vi "anodicFitTest.vi"() -> ()   [LabVIEW 2018]
uses:
  <vilib>/Utility/file.llb/Read Delimited Spreadsheet (DBL).vi
panel:
  in  "iCorr":dbl=0.009000000000000001 step=0.001 format="%#_13g"
  out "return":dbl
  out "anodicElements":i32=115
  out "eCorr":dbl=-0.202
  out "intersects":i32
  out "anodicFitCoeffs":dbl[](array[numeric])=[-0.23570360753794362, -0.007154949128379092, 0.0, 0.0]
  out "anodicTraceCoeffs":dbl[](array[numeric])=[-0.21186227610841735, 0.0007290916455038351, 0.0, 0.0]
  in  "y2":dbl=-0.22000000000000003 step=0.01 format="%#_13g"
  in  "yData Filename":string="yData2"
  in  "xData Filename":string="xData2"
  out "error out":errorcluster
  out "MEASUREMENT":cluster{"XCoords":dbl[], "YCoords":dbl[]}[](graph)=[{"XCoords"=[1.108281, 0.885344, 0.732926, 0.625224, 0.543485, 0.479698, 0.42809, 0.384497, 0.350199, 0.321029, 0.296828, 0.273749, 0.255959, 0.241054, 0.227752, 0.21493, 0.202269, 0.193774, 0.184158, 0.177427, 0.168131, 0.162041, 0.156591, 0.150822, 0.143289, 0.138641, 0.133833, 0.129666, 0.124858, 0.119889, 0.116844, 0.112998, 0.109952, 0.104824, 0.103221, 0.099375, 0.09649, 0.093765, 0.09072, 0.088957, 0.086072, 0.083508, 0.080302, 0.07918, 0.077097, 0.074853, 0.071968, 0.069564, 0.068122, 0.066198, 0.064596, 0.06139, 0.060749, 0.059147, 0.056903, 0.055621, 0.053377, 0.052095, 0.050812, 0.049049, 0.045684, 0.044722, 0.044081, 0.04344, 0.040074, 0.038952, 0.037991, 0.036709, 0.036709, 0.033824, 0.03142, 0.0319, 0.029817, 0.027733, 0.027092, 0.02565, 0.02581, 0.022605, 0.021323, 0.021323, 0.019079, 0.019399, 0.016514, 0.015553, 0.014591, 0.012988, 0.012988, 0.010745, 0.009783, 0.008661, 0.009142, 0.006417, 0.006898, 0.005295, 0.002731, 0.00209, 7e-06, 0.000487, 0.000635, 0.001756, 0.00368, 0.004641, 0.005763, 0.006404, 0.007526, 0.008167, 0.008808, 0.008969, 0.010892, 0.012975, 0.012655, 0.013616, 0.013616, 0.016501, 0.018104, 0.017463, 0.019386, 0.020668, 0.023072, 0.023714, 0.023714, 0.026278, 0.0274, 0.028041, 0.028682, 0.029964, 0.029964, 0.031727, 0.032208, 0.034452, 0.034452, 0.034452, 0.036535, 0.036696, 0.037657, 0.038939, 0.040702, 0.040863, 0.042305, 0.042145, 0.04519, 0.04535, 0.046632, 0.046632, 0.049036, 0.048876, 0.049838, 0.050158, 0.05144, 0.053364, 0.053684, 0.055447, 0.054646, 0.05689, 0.057531, 0.058172, 0.059454, 0.059775, 0.061057, 0.062659, 0.06298, 0.064262, 0.066185, 0.066826, 0.067468, 0.068429, 0.06907, 0.070352, 0.071635, 0.071474, 0.073237, 0.07468, 0.073878, 0.074359, 0.076763, 0.075802, 0.079328, 0.079648, 0.079969, 0.081251, 0.082533, 0.083815, 0.084456, 0.085738, 0.087822, 0.087982, 0.089745, 0.089905, 0.090547, 0.09247, 0.093431, 0.094874, 0.095996, 0.097919, 0.09824, 0.09856, 0.099201, 0.099201, 0.100964, 0.099842, 0.101445, 0.103368, 0.105292, 0.10465, 0.105933, 0.104971, 0.106894, 0.109138, 0.109459, 0.109459, 0.111382], "YCoords"=[-0.298, -0.297, -0.296, -0.295, -0.294, -0.293, -0.292, -0.291, -0.29, -0.289, -0.288, -0.287, -0.286, -0.285, -0.284, -0.283, -0.282, -0.281, -0.28, -0.279, -0.278, -0.277, -0.276, -0.275, -0.274, -0.273, -0.272, -0.271, -0.27, -0.269, -0.268, -0.267, -0.266, -0.265, -0.264, -0.263, -0.262, -0.261, -0.26, -0.259, -0.258, -0.257, -0.256, -0.255, -0.254, -0.253, -0.252, -0.251, -0.25, -0.249, -0.248, -0.247, -0.246, -0.245, -0.244, -0.243, -0.242, -0.241, -0.24, -0.239, -0.238, -0.237, -0.236, -0.235, -0.234, -0.233, -0.232, -0.231, -0.23, -0.229, -0.228, -0.227, -0.226, -0.225, -0.224, -0.223, -0.222, -0.221, -0.22, -0.219, -0.218, -0.217, -0.216, -0.215, -0.214, -0.213, -0.212, -0.211, -0.21, -0.209, -0.208, -0.207, -0.206, -0.205, -0.204, -0.203, -0.202, -0.201, -0.2, -0.199, -0.198, -0.197, -0.196, -0.195, -0.194, -0.193, -0.192, -0.191, -0.19, -0.189, -0.188, -0.187, -0.186, -0.185, -0.184, -0.183, -0.182, -0.181, -0.18, -0.179, -0.178, -0.177, -0.176, -0.175, -0.174, -0.173, -0.172, -0.171, -0.17, -0.169, -0.168, -0.167, -0.166, -0.165, -0.164, -0.163, -0.162, -0.161, -0.16, -0.159, -0.158, -0.157, -0.156, -0.155, -0.154, -0.153, -0.152, -0.151, -0.15, -0.149, -0.148, -0.147, -0.146, -0.145, -0.144, -0.143, -0.142, -0.141, -0.14, -0.139, -0.138, -0.137, -0.136, -0.135, -0.134, -0.133, -0.132, -0.131, -0.13, -0.129, -0.128, -0.127, -0.126, -0.125, -0.124, -0.123, -0.122, -0.121, -0.12, -0.119, -0.118, -0.117, -0.116, -0.115, -0.114, -0.113, -0.112, -0.111, -0.11, -0.109, -0.108, -0.107, -0.106, -0.105, -0.104, -0.103, -0.102, -0.101, -0.1, -0.099, -0.098, -0.097, -0.096, -0.095, -0.094, -0.093, -0.092, -0.091, -0.09, -0.089, -0.088]}, {"XCoords"=[7e-06, 0.0009671052631578947, 0.0019272105263157895, 0.002887315789473684, 0.003847421052631579, 0.004807526315789474, 0.005767631578947368, 0.006727736842105263, 0.007687842105263158, 0.008647947368421052, 0.009608052631578948, 0.010568157894736842, 0.011528263157894736, 0.012488368421052632, 0.013448473684210526, 0.014408578947368422, 0.015368684210526316, 0.01632878947368421, 0.017288894736842104, 0.018249, 0.019209105263157895, 0.02016921052631579, 0.021129315789473684, 0.022089421052631578, 0.02304952631578947, 0.02400963157894737, 0.024969736842105263, 0.025929842105263157, 0.02688994736842105, 0.027850052631578946, 0.028810157894736843, 0.029770263157894737, 0.03073036842105263, 0.031690473684210525, 0.03265057894736842, 0.03361068421052631, 0.03457078947368421, 0.0355308947368421, 0.036491, 0.0374511052631579, 0.03841121052631579, 0.039371315789473685, 0.04033142105263158, 0.04129152631578947, 0.04225163157894737, 0.04321173684210526, 0.044171842105263155, 0.04513194736842105, 0.04609205263157894, 0.047052157894736844, 0.04801226315789474, 0.04897236842105263, 0.04993247368421053, 0.05089257894736842, 0.051852684210526315, 0.05281278947368421, 0.0537728947368421, 0.054733, 0.05569310526315789, 0.05665321052631579, 0.057613315789473686, 0.05857342105263158, 0.059533526315789474, 0.06049363157894737, 0.06145373684210526, 0.062413842105263156, 0.06337394736842106, 0.06433405263157894, 0.06529415789473685, 0.06625426315789473, 0.06721436842105263, 0.06817447368421052, 0.06913457894736842, 0.07009468421052631, 0.07105478947368421, 0.07201489473684211, 0.072975, 0.0739351052631579, 0.07489521052631579, 0.07585531578947369, 0.07681542105263157, 0.07777552631578948, 0.07873563157894736, 0.07969573684210526, 0.08065584210526315, 0.08161594736842105, 0.08257605263157895, 0.08353615789473684, 0.08449626315789474, 0.08545636842105263, 0.08641647368421053, 0.08737657894736842, 0.08833668421052632, 0.0892967894736842, 0.0902568947368421, 0.09121699999999999, 0.0921771052631579, 0.0931372105263158, 0.09409731578947368, 0.09505742105263158, 0.09601752631578947, 0.09697763157894737, 0.09793773684210526, 0.09889784210526316, 0.09985794736842105, 0.10081805263157895, 0.10177815789473683, 0.10273826315789474, 0.10369836842105264, 0.10465847368421052, 0.10561857894736842, 0.10657868421052631, 0.10753878947368421, 0.1084988947368421, 0.109459], "YCoords"=[-0.2118515633561114, -0.21038734537997142, -0.20893324738712393, -0.20748919943302277, -0.2060551320565454, -0.20463097627665186, -0.20321666358906648, -0.20181212596298284, -0.2004172958377913, -0.19903210611982933, -0.19765649017915402, -0.1962903818463372, -0.1949337154092826, -0.1935864256100648, -0.19224844764179053, -0.190919717145481, -0.1896001702069764, -0.18828974335386134, -0.18698837355241185, -0.18569599820456326, -0.1844125551448992, -0.18313798263766132, -0.18187221937377962, -0.18061520446792345, -0.1793668774555729, -0.17812717829011016, -0.1768960473399314, -0.17567342538557815, -0.17445925361688902, -0.17325347363017057, -0.1720560274253882, -0.1708668574033761, -0.1696859063630667, -0.16851311749873926, -0.1673484343972873, -0.16619180103550513, -0.16504316177739298, -0.16390246137148085, -0.16276964494817078, -0.16164465801709768, -0.16052744646450798, -0.15941795655065694, -0.15831613490722352, -0.15722192853474326, -0.1561352848000591, -0.1550561514337894, -0.15398447652781383, -0.15292020853277652, -0.15186329625560635, -0.1508136888570546, -0.14977133584924937, -0.14873618709326716, -0.14770819279672096, -0.14668730351136525, -0.14567347013071746, -0.14466664388769587, -0.14366677635227373, -0.14267381942914978, -0.14168772535543483, -0.14070844669835417, -0.13973593635296605, -0.13877014753989586, -0.13781103380308588, -0.1368585490075608, -0.13591264733720845, -0.13497328329257596, -0.13404041168868122, -0.13311398765283938, -0.13219396662250443, -0.13128030434312557, -0.13037295686601863, -0.12947188054625192, -0.128577032040547, -0.12768836830519362, -0.12680584659397937, -0.1259294244561335, -0.1250590597342849, -0.12419471056243434, -0.12333633536394058, -0.12248389284952048, -0.121637342015263, -0.12079664214065668, -0.11996175278663108, -0.11913263379361148, -0.11830924527958722, -0.11749154763819321, -0.1166795015368049, -0.11587306791464624, -0.11507220798091085, -0.11427688321289609, -0.11348705535414998, -0.11270268641263116, -0.11192373865888129, -0.11115017462421023, -0.11038195709889372, -0.10961904913038356, -0.10886141402153011, -0.10810901532881713, -0.10736181686060871, -0.10661978267540845, -0.10588287708013064, -0.10515106462838328, -0.10442431011876313, -0.10370257859316238, -0.10298583533508722, -0.10227404586798779, -0.10156717595359992, -0.1008651915902981, -0.10016805901146006, -0.09947574468384243, -0.0987882153059678, -0.09810543780652288, -0.09742737934276763, -0.09675400729895556, -0.09608528928476477]}, {"XCoords"=[0.008999999999999998, 0.010975669036994953, 0.012951338073989908, 0.014927007110984863, 0.016902676147979818, 0.018878345184974773, 0.020854014221969728, 0.022829683258964683, 0.024805352295959638, 0.026781021332954593, 0.028756690369949548, 0.030732359406944503, 0.032708028443939455, 0.03468369748093442, 0.036659366517929365, 0.03863503555492433, 0.040610704591919275, 0.04258637362891424, 0.044562042665909185, 0.04653771170290415, 0.048513380739899095, 0.05048904977689406, 0.052464718813889005, 0.05444038785088397, 0.056416056887878915, 0.05839172592487388, 0.060367394961868825, 0.06234306399886379, 0.06431873303585874, 0.0662944020728537, 0.06827007110984865, 0.07024574014684361, 0.07222140918383856, 0.07419707822083352, 0.07617274725782847, 0.07814841629482343, 0.08012408533181838, 0.08209975436881334, 0.08407542340580829, 0.08605109244280325, 0.0880267614797982, 0.09000243051679316, 0.0919780995537881, 0.09395376859078307, 0.09592943762777802, 0.09790510666477298, 0.09988077570176793, 0.10185644473876289, 0.10383211377575784, 0.1058077828127528], "YCoords"=[-0.2019999999999992, -0.20341994501588523, -0.2046042192579689, -0.20562002900118723, -0.20650938797086996, -0.20730032142205354, -0.20801246031008225, -0.20866009144773573, -0.2092539369261141, -0.2098022495062892, -0.21031151711473367, -0.21078693274037513, -0.21123271765386534, -0.21165234967764396, -0.21204872812831538, -0.21242429541001304, -0.21278112824994538, -0.21312100724039493, -0.21344547059700883, -0.2137558562462068, -0.21405333515608854, -0.21433893800998408, -0.21461357675719273, -0.21487806217800662, -0.2151331183161254, -0.21537939442585335, -0.21561747493056393, -0.215847887776919, -0.21607111148530825, -0.21628758113330132, -0.2164976934602025, -0.21670181124321622, -0.21690026706649446, -0.21709336658141623, -0.21728139133834884, -0.21746460125575068, -0.21764323678096076, -0.2178175207877494, -0.2179876602482001, -0.21815384771038077, -0.21831626260826337, -0.21847507242623784, -0.2186304337371692, -0.21878249313012674, -0.21893138804156426, -0.2190772475017629, -0.2192201928066972, -0.21936033812408945, -0.21949779104124104, -0.21963265306122537]}]
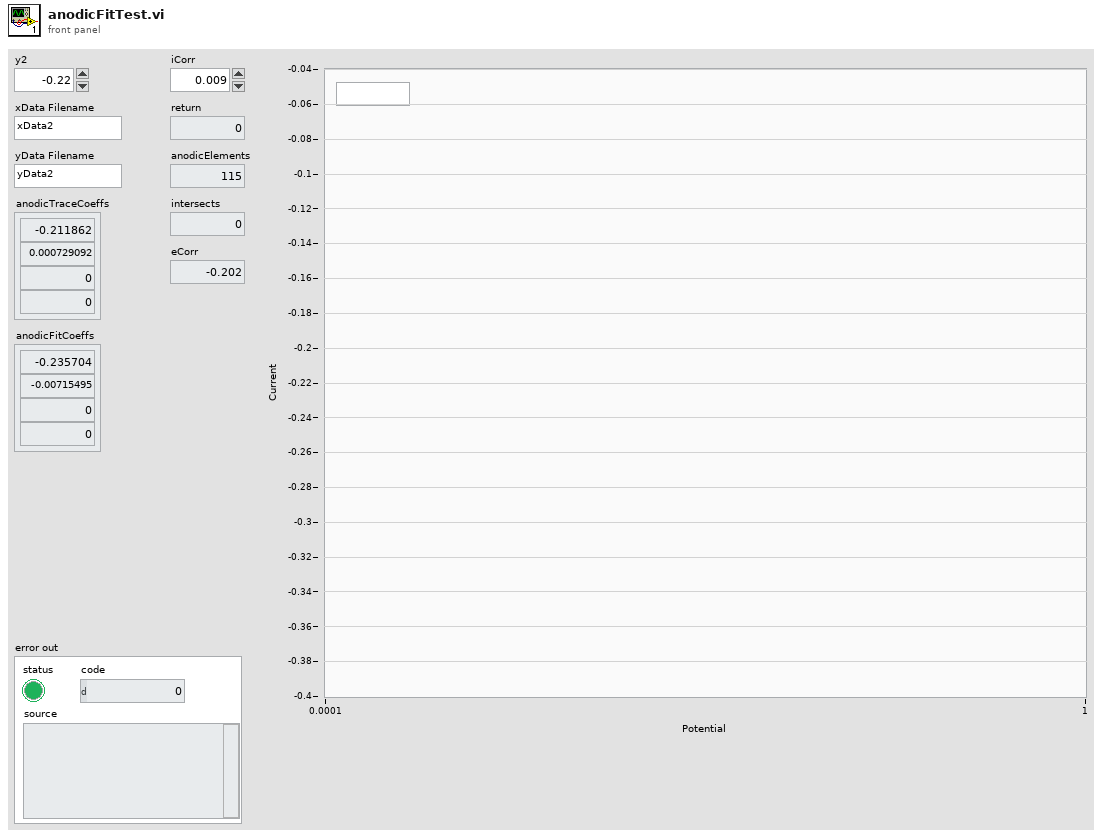
[diagram p1: front panel]
types:
  T1 = cluster{"AnodicTrace":cluster{"XCoords":dbl[], "YCoords":dbl[]}, "AnodicFit":cluster{"XCoords":dbl[], "YCoords":dbl[]}}
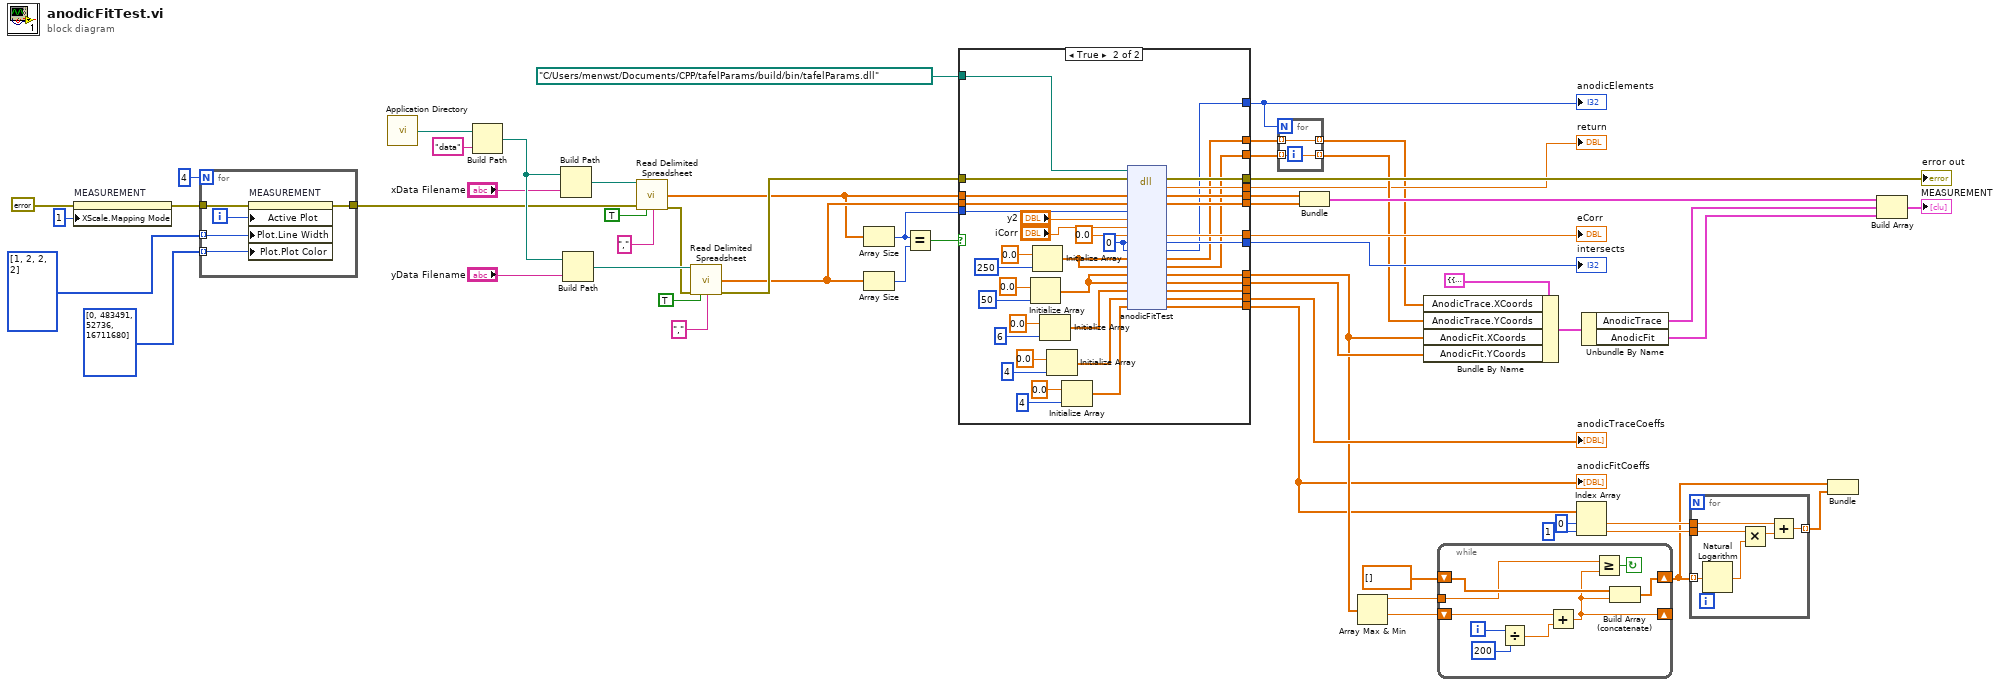
[diagram p0: block diagram]
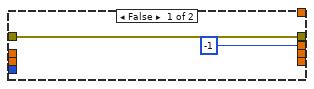
[diagram p2: hidden frame]
diagram:
  n1 = property on="MEASUREMENT" class="XYGraph (strict)"(error in=errorcluster {"status"=FALSE, "code"=0, "source"=""} ("error out"), "XScale.Mapping Mode"=u8 1 ("X Scale.Mapping Mode")) -> (error out=w31:errorcluster)  [unwired: 1 in, 1 out]
  n2 = for {
    N: 4 -> [_]
    tunnel: w31 -> [w60]
    tunnel: [w59] -> w30
    tunnel: u32[] [0, 483491, 52736, 16711680] -> [w58] mode=indexing
    tunnel: i32[] [1, 2, 2, 2] -> [w57] mode=indexing
    i -> [w61]
    n3 = property on="MEASUREMENT" class="XYGraph (strict)"(error in=w60, "Active Plot"=w61, "Plot.Line Width"=w57, "Plot.Plot Color"=w58) -> (error out=w59:errorcluster)  [unwired: 1 in, 1 out]
  }
  n4 = call <vilib>:"Application Directory.vi"() -> ("Application Directory"=w52:path)
  n5 = Build Path(base path=w52, name or relative path="data") -> (appended path=w50:path)
  n6 = Build Path(base path=w50, name or relative path="xData Filename") -> (appended path=w47:path)
  n7 = Build Path(base path=w50, name or relative path="yData Filename") -> (appended path=w46:path)
  n8 = call-poly <vilib>:"Read Delimited Spreadsheet.vi"("file path (dialog if empty)"=w47, "error in (no error)"=w30, "transpose? (F)"=TRUE, "delimiter (\\t)"="," ("delimiter (\\t)")) -> ("first row"=w24:dbl[], "error out"=w44:errorcluster)  [unwired: 6 in, 4 out]
  n9 = call-poly <vilib>:"Read Delimited Spreadsheet.vi"("file path (dialog if empty)"=w46, "error in (no error)"=w44, "transpose? (F)"=TRUE, "delimiter (\\t)"="," ("delimiter (\\t)")) -> ("first row"=w25:dbl[], "error out"=w43:errorcluster)  [unwired: 6 in, 4 out]
  n10 = Array Size(array=w24) -> (size(s)=w37:i32)
  n11 = Array Size(array=w25) -> (size(s)=w42:i32)
  n12 = Equal?(x=w37, y=w42) -> (x = y?=w41:bool)
  n13 = case shown="True" w41 {
    tunnel: [w62 w101] -> w23
    tunnel: [-1 ("return type") w100] -> w15
    tunnel: w25 -> [_ w94]
    tunnel: w24 -> [_ w95]
    tunnel: w43 -> [w62 w99]
    tunnel: path "C:/Users/menwst/Documents/CPP/tafelParams/build/bin/tafelParams.dll" ("path in") -> [_ w98]
    tunnel: [_ w91] -> w27
    tunnel: [_ w90] -> w26
    tunnel: w37 -> [_ w93]
    tunnel: [_ w77] -> w10
    tunnel: [_ w76] -> w22
    tunnel: [_ w75] -> w14
    tunnel: [_ w74] -> w7
    tunnel: [_ w70] -> _
    tunnel: [_ w69] -> w21
    tunnel: [_ w68] -> w20
    tunnel: [_ w67] -> w19
    tunnel: [_ w66] -> w18
    tunnel: [_ w65] -> w17
    frame False {
    }
    frame True {
      w88 = 0 ("intersects")
      n14 = Initialize Array(0.0 ("element"), 50 ("xnumRows")) -> (w84:dbl[])
      n15 = Initialize Array(0.0 ("element"), 250 ("xnumRows")) -> (w87:dbl[])
      n16 = Initialize Array(0.0 ("element"), 6 ("xnumRows")) -> (w71:dbl[])
      n17 = Initialize Array(0.0 ("element"), 4 ("xnumRows")) -> (w81:dbl[])
      n18 = Initialize Array(0.0 ("element"), 4 ("xnumRows")) -> (w78:dbl[])
      n19 = dll-call lib="C:/Users/menwst/Documents/CPP/tafelParams/build/bin/tafelParams.dll" fn="anodicFitTest"(path in=w98, error in=w99, "xdata"=w95, "ydata"=w94, "numRows"=w93, "y2"="y2", "iCorr"="iCorr", "eCorr"=0.0 ("element"), "intersects"=w88, "anodicElements"=w88, "xAnodicTrace"=w87, "yAnodicTrace"=w87, "xAnodicFit"=w84, "yAnodicFit"=w84, "solutions"=w71, "anodicTraceCoeffs"=w81, "anodicFitCoeffss"=w78) -> (error out=w101:errorcluster, "return type"=w100:dbl, "xdata"=w91:dbl[], "ydata"=w90:dbl[], "eCorr"=w68:dbl, "intersects"=w69:i32, "anodicElements"=w67:i32, "xAnodicTrace"=w66:dbl[], "yAnodicTrace"=w65:dbl[], "xAnodicFit"=w77:dbl[], "yAnodicFit"=w76:dbl[], "solutions"=w70:dbl[], "anodicTraceCoeffs"=w75:dbl[], "anodicFitCoeffss"=w74:dbl[])  [unwired: 4 in, 1 out]
    }
  }
  "error out" <- w23
  "anodicTraceCoeffs" <- w14
  "anodicFitCoeffs" <- w7
  "intersects" <- w21
  "eCorr" <- w20
  "anodicElements" <- w19
  "return" <- w15
  n20 = for {
    N: w19 -> [_]
    tunnel: w18 -> [w103] mode=indexing
    tunnel: w17 -> [w102] mode=indexing
    tunnel: [w103] -> w13 mode=indexing
    tunnel: [w102] -> w16 mode=indexing
  }
  n21 = Bundle("xdata"=w27, "ydata"=w26) -> (w33:cluster{"xdata":dbl[], "ydata":dbl[]})  [unwired: 1 in]
  n22 = Array Max & Min(array=w10) -> (max value=w9:dbl, min value=w8:dbl)  [unwired: 2 out]
  n23 = Bundle By Name(cluster=T1 {"AnodicTrace"={"XCoords"=[], "YCoords"=[]}, "AnodicFit"={"XCoords"=[], "YCoords"=[]}} ("Fit Coords"), "AnodicTrace.XCoords"=w13, "AnodicTrace.YCoords"=w16, "AnodicFit.XCoords"=w10, "AnodicFit.YCoords"=w22) -> (w39:T1)
  n24 = while {
    shift-right: [w112] -> w1
    shift-left: dbl[] [] -> [w111]
    shift-right: [w106] -> _
    shift-left: w8 -> [w110]
    tunnel: w9 -> [w105]
    i -> [w107]
    stop <- w109 continue-if-true
    n25 = Divide(x=w107, y=200) -> (x/y=w104:dbl)
    n26 = Add(x=w110, y=w104) -> (x+y=w106:dbl)
    n27 = Greater Or Equal?(x=w105, y=w106) -> (x >= y?=w109:bool)
    n28 = Build Array (concatenate)(w111, w106) -> (w112:dbl[])
  }
  n29 = Index Array(array=w7, index #1=0 ("index"), index #2=1 ("index")) -> (element #1=w4:dbl, element #2=w3:dbl)
  n30 = Unbundle By Name(w39) -> ("AnodicTrace"=w38:cluster{"XCoords":dbl[], "YCoords":dbl[]}, "AnodicFit"=w12:cluster{"XCoords":dbl[], "YCoords":dbl[]})
  n31 = for {
    tunnel: w1 -> [w118] mode=indexing
    tunnel: w4 -> [w115]
    tunnel: w3 -> [w117]
    tunnel: [w113] -> w2 mode=indexing
    n32 = Natural Logarithm(1:w118) -> (0:w116:dbl)
    n33 = Multiply(x=w117, y=w116) -> (x*y=w114:dbl)
    n34 = Add(x=w115, y=w114) -> (x+y=w113:dbl)
  }
  n35 = Bundle(w1, w2) -> ()  [unwired: 1 in, 1 out]
  n36 = Build Array(w33, w38, w12) -> (→"MEASUREMENT":cluster{"XCoords":dbl[], "YCoords":dbl[]}[])
